vi "Telemetry Transmitter.vi"   [LabVIEW 2021]
doc: "This VI reads in data from the telemetry handler and redistributes it to all the various transmission protocols."
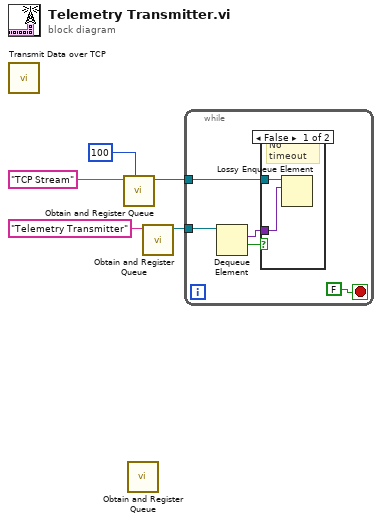
[diagram p0: block diagram]
diagram:
  n1 = call "Transmit Data over TCP.vi"() -> ()  [unwired: 12 in]
  n2 = call "Obtain and Register Queue.vi"("max queue size (-1, unlimited)"=100, "Queue Name (unnamed)"="TCP Stream" ("name (unnamed)")) -> ("Queue Reference"=w5:refnum<queue>)  [unwired: 8 in, 1 out]
  n3 = call "Obtain and Register Queue.vi"() -> ()  [unwired: 10 in, 2 out]
  n4 = call "Obtain and Register Queue.vi"("Queue Name (unnamed)"="Telemetry Transmitter" ("name (unnamed)")) -> ("Queue Reference"=w4:refnum<queue>)  [unwired: 9 in, 1 out]
  n5 = while {
    tunnel: w4 -> [w10]
    tunnel: w5 -> [w8]
    stop <- FALSE stop-if-true
    n6 = Dequeue Element(queue=w10) -> (element=w7:variant, timed out?=w6:bool)  [unwired: 2 in, 2 out]
    n7 = case shown="False" w6 {
      tunnel: w8 -> [w12 _]
      tunnel: w7 -> [w11 _]
      frame False {
        # "No timeout"
        n8 = Lossy Enqueue Element(queue=w12, element=w11) -> ()  [unwired: 1 in, 4 out]
      }
      frame True {
        # "Timed out"
      }
    }
  }
